vi "gfitsio-movabs-hdu.vi"(7 "hdunum":i32, 8 "error in (no error)":errorcluster, 11 "gfits refnum":T2) -> (0 "error out":errorcluster, 2 "hdutype":T1 items=["ANY_HDU"=-1, "IMAGE_HDU"=0, "ASCII_TBL"=1, "BINARY_TBL"=2], 3 "dup gfits refnum":T2)   [LabVIEW 2019, in "gfitsio.lvlib"]
doc: "Move to a different HDU in the file. HDU number (starting with 1 for the primary array) specifies the absolute index of the HDU to move to in the FITS file. <B>hdutype</B> contains the type of the destination HDU."
uses:
  gfitsio.lvlib
  gfitsio-refnum.ctl
  cfitsio-hdutypes.ctl
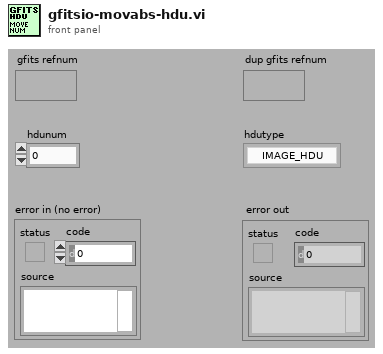
[diagram p1: front panel]
types:
  T1 = typedef "gfitsio.lvlib/cfitsio-hdutypes.ctl" = i32
  T2 = typedef "gfitsio.lvlib/gfitsio-refnum.ctl" = refnum<k1>
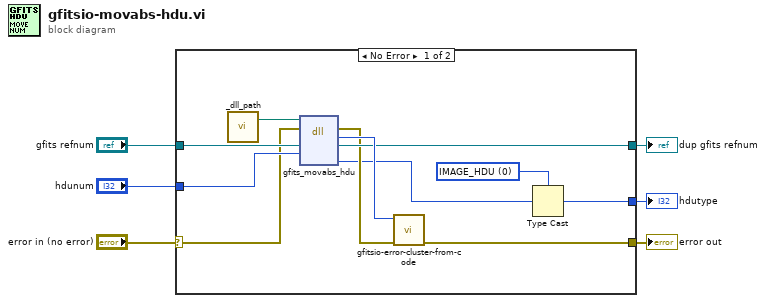
[diagram p0: block diagram]
diagram:
  n1 = case shown="No Error" "error in (no error)" {
    selector: "error in (no error)" -> [w12 w19]
    tunnel: [w16 w19] -> w6
    tunnel: "hdunum" -> [w15 _]
    tunnel: [w14 w18] -> w3
    tunnel: "gfits refnum" -> [w13 w18]
    tunnel: [w9 _] -> w1
    frame No Error {
      w8 = T1 0 items=["ANY_HDU"=-1, "IMAGE_HDU"=0, "ASCII_TBL"=1, "BINARY_TBL"=2] ("hdutype")
      n2 = call "_dll_path.vi"() -> ("Path"=w7:path)  [unwired: 1 in]
      n3 = dll-call lib="?" fn="gfits_movabs_hdu"(path in=w7, error in=w12, "refnum"=w13, "hdunum"=w15) -> (error out=w11:errorcluster, "return type"=w17:i32, "refnum"=w14:T2, "hdutype"=w10:i32)  [unwired: 2 in, 2 out]
      n4 = call "gfitsio-error-cluster-from-code.vi"("error in (no error)"=w11, "error code"=w17) -> ("error out"=w16:errorcluster)  [unwired: 9 out]
      n5 = Type Cast(type=w8, x=w10) -> (*(type *) &x=w9:T1)
    }
    frame Error {
    }
  }
  "error out" <- w6
  "dup gfits refnum" <- w3
  "hdutype" <- w1
